vi "Log Error.vi"(8 "error in":errorcluster, 11 "Module Data In":refnum<class "Rename.lvclass">) -> (0 "error out":errorcluster, 3 "Module Data Out":refnum<class "Rename.lvclass">)   [LabVIEW 2015, in "Generic Module Library.lvlib" / "Template G_Module.lvlib"]
uses:
  Template G_Module.lvlib
  Module Class/Rename.lvclass
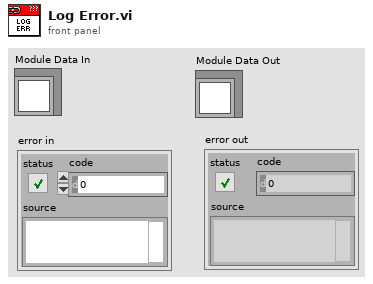
[diagram p1: front panel]
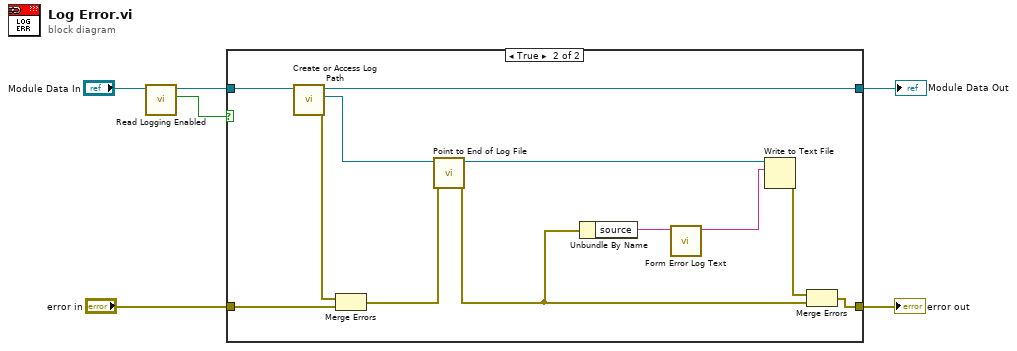
[diagram p0: block diagram]
diagram:
  n1 = call-dynamic "Read Logging Enabled.vi"("Rename in"="Module Data In") -> ("Logging Enabled"=w1:bool, "Rename out"=w2:refnum<class "Rename.lvclass">)  [unwired: 8 in, 1 out]
  n2 = case shown="True" w1 {
    tunnel: [w7 w20] -> w6
    tunnel: "error in" -> [w7 w19]
    tunnel: [w8 w17] -> w4
    tunnel: w2 -> [w8 w9]
    frame False {
    }
    frame True {
      n3 = call "Create or Access Log Path.vi"("Module Data In"=w9) -> ("error out"=w18:errorcluster, "Log Refnum Out"=w13:refnum<file>, "Module Data Out"=w17:refnum<class "Rename.lvclass">)  [unwired: 7 in, 1 out]
      n4 = Merge Errors(w18, w19) -> (w11:errorcluster)
      n5 = call "Point to End of Log File.vi"("error in (no error)"=w11, "Byte Stream File in"=w13) -> ("error out"=w10:errorcluster, "Byte Stream File out"=w12:refnum<file>)  [unwired: 8 in]
      n6 = Unbundle By Name(w10) -> ("source"=w15:string)
      n7 = call "Form Error Log Text.vi"("Error Source Input"=w15) -> ("String to Write"=w16:string)  [unwired: 10 in]
      n8 = Write to Text File(file (use dialog)=w12, text=w16) -> (error out=w14:errorcluster)  [unwired: 2 in, 2 out]
      n9 = Merge Errors(w14, w10) -> (w20:errorcluster)
    }
  }
  "error out" <- w6
  "Module Data Out" <- w4
